vi "TestHighScores.vi"() -> ()   [LabVIEW 2019]
uses:
  TextDisplay Class.lvclass
panel:
  out "String":string
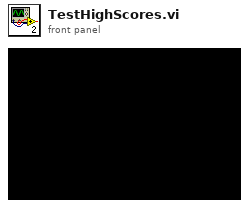
[diagram p1: front panel]
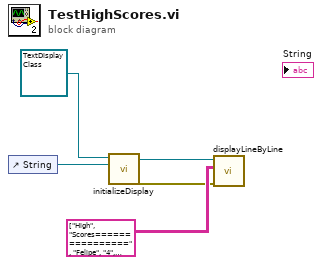
[diagram p0: block diagram]
diagram:
  n1 = control-ref of="String"() -> (w1:refnum<vi>)
  n2 = call "initializeDisplay.vi"("stringControlRefnum"=w1, "TextDisplay Class in"=refnum<class "TextDisplay Class.lvclass"> refnum) -> ("error out"=w3:errorcluster, "TextDisplay Class out"=w4:refnum<class "TextDisplay Class.lvclass">)  [unwired: 8 in]
  n3 = call "displayLineByLine.vi"("error in (no error)"=w3, "scoreLog"=string[][] [["High", "Scores"], ["=========", "========="], ["Felipe", "4"], ["Lincoln", "6"], ["Plinio", "5"], ["Ligia", "9"], ["Belle", "4"]], "TextDisplay Class in"=w4) -> ()  [unwired: 7 in, 2 out]
